vi "Data Format Operations.vi"(0 "VISA resource name":refnum<visa-resource-name>, 5 "Data Format (0:Ascii)":i32(ring) items=["Ascii", "Real", "Integer"], 7 "Length (0:0)":i32(ring) items=["0", "32"], 9 "Byte Order (0:Normal)":i32(ring) items=["Normal", "Swap"], 11 "error in (no error)":errorcluster) -> (4 "VISA resource name out":refnum<visa-resource-name>, 15 "error out":errorcluster)   [LabVIEW 2020, in "Anritsu Signal Analyzer Series.lvlib"]
doc: "Sets the format of the data that is read."
uses:
  Anritsu Signal Analyzer Series.lvlib
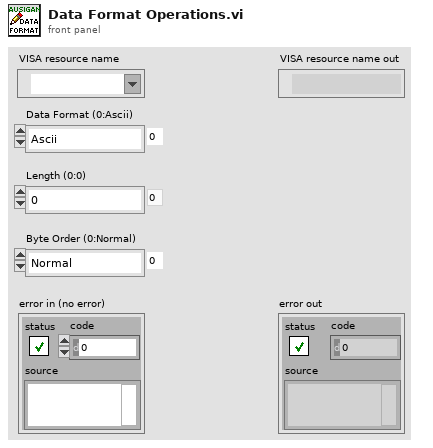
[diagram p1: front panel]
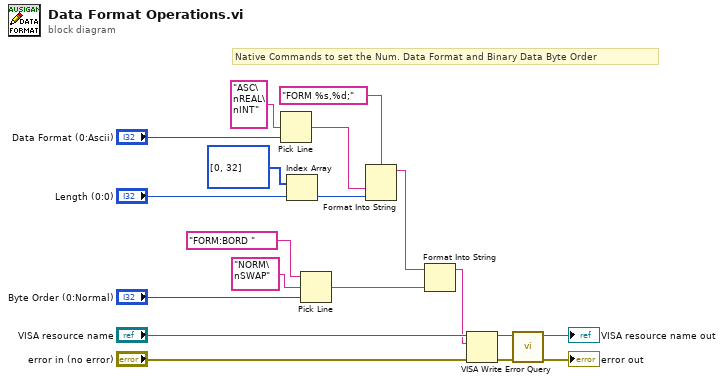
[diagram p0: block diagram]
diagram:
  # "Native Commands to set the Num. Data Format and Binary Data Byte Order"
  n1 = Pick Line(multi-line string="ASC\nREAL\nINT" ("string"), line index="Data Format (0:Ascii)") -> (output string=w11:string)  [unwired: 1 in]
  n2 = Index Array(array=i32[] [0, 32], index="Length (0:0)") -> (element=w6:i32)
  n3 = Pick Line(string ("")="FORM:BORD " ("_CommandSet"), multi-line string="NORM\nSWAP" ("string"), line index="Byte Order (0:Normal)") -> (output string=w2:string)
  n4 = Format Into String(format string="FORM %s,%d;" ("形式文字列"), w11, w6) -> (resulting string=w1:string)  [unwired: 2 in, 1 out]
  n5 = Format Into String(initial string=w1, w2) -> (resulting string=w8:string)  [unwired: 2 in, 1 out]
  n6 = VISA Write(VISA resource name="VISA resource name", write buffer=w8, error in (no error)="error in (no error)") -> (VISA resource name out=w14:refnum<visa-resource-name>, error out=w13:errorcluster)  [unwired: 1 out]
  n7 = call "Error Query.vi"("error in (no error)"=w13, "VISA resource name"=w14) -> ("error out"=→"error out":errorcluster, "VISA resource name out"=→"VISA resource name out":refnum<visa-resource-name>)  [unwired: 6 in, 2 out]
